vi "RT Main.vi"() -> ()   [LabVIEW 2018]
uses:
  <vilib>/Utility/RT CPU Load.ctl
  <vilib>/FPGAPlugInAG/cRIO-9056/niLvFpga_Open_cRIO-9056.vi
  <vilib>/FPGAPlugInAG/cRIO-9056/niLvFpga_Close_cRIO-9056.vi
  <vilib>/rvi/interface/nirviOpenFPGA/nirviOpenFPGA.xnode
  Type Defs/FPGA reference.ctl
  FPGA Bitfiles/CompressorRigV2_CompressorFPGA_FPGAMainV3_7sPRekuravM.lvbitx
  <vilib>/rvi/interface/nirviCloseFPGA/nirviCloseFPGA.xnode
  <vilib>/NI_Real-Time Target Support.lvlib
panel:
  out "CPU loads":T1[](array[typedef]) {"ISR (%)" format="%#.2f"; "Idle (%)" format="%#.2f"; "Background (%)" format="%#.2f"; "Normal (%)" format="%#.2f"; "Above Normal (%)" format="%#.2f"; "High (%)" format="%#.2g"; "Timed Structures (%)" format="%#.2g"; "Time Critical (%)" format="%#.2g"; "Total (%)" format="%#.2g"}
  in  "Stop display loop":bool
  in  "Queue":enum16{"Message", "Comms", "Data"}(ring)=enum."Data"
  in  "show":bool
  out "messages":string[](array[string])
  out "queue sizes":i32[](array[numeric])
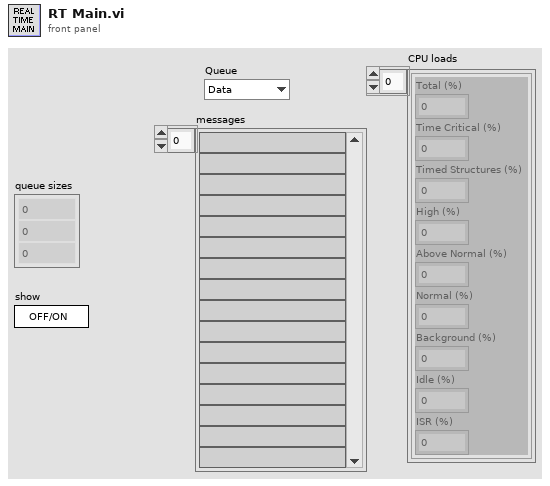
[diagram p1: front panel]
types:
  T1 = typedef "NI_Real-Time Target Support.lvlib/RT CPU Load.ctl" = cluster{"Total (%)":dbl, "Time Critical (%)":dbl, "Timed Structures (%)":dbl, "High (%)":dbl, "Above Normal (%)":dbl, "Normal (%)":dbl, "Background (%)":dbl, "Idle (%)":dbl, "ISR (%)":dbl}
  T2 = typedef "FPGA reference.ctl" = refnum<k20>
  T3 = typedef "Message loop data.ctl" = cluster{"Parameters":cluster{"FPGA Ref":T2, "configID":u32, "activeChannels":cluster{"index":u16, "name":string}[]}, "Variables":cluster{"RT Status":T4, "watchdog":timestamp, "limitsEnabled":bool, "Interlocks":cluster{"gearboxOil":bool, "bearingOil":bool, "gearboxAir":bool}}}
  T4 = typedef "RT Status.ctl" = cluster{"Comms loop":bool, "scheduler loop":bool, "data process loop":bool, "FIFO loop":bool, "Command Stream":bool, "Error Stream":bool, "FPGA FIFO":bool, "Data Stream":bool}
  T5 = typedef "Analogue loop data.ctl" = cluster{"Params":cluster{"FPGA ref":T2, "Total Channels":u32}, "Variables":cluster{"FIFO wait counter":u16, "FIFO read trigger":u32}}
  T6 = typedef "comms data.ctl" = cluster{"Parameters":cluster{"error writer name":string, "command reader name":string, "error buffer size":i32, "command buffer size":i32, "scanivalveIP":string, "scanivalvePeriod":u16}, "Variables":cluster{"listen schedule":u32, "incident buffer":T7[], "command stream":refnum<k21>, "error stream":refnum<k21>, "waiting for command stream connect":bool, "waiting for error stream connect":bool, "scanivalve connection":refnum<k5>, "scanivalveScheduleID":u32, "activeScanivalvePorts":i32[], "channelCount":i16}, "scanivalveConfig":T8}
  T7 = typedef "generic incident.ctl" = cluster{"timestamp":timestamp, "type":string, "Variant":variant}
  T8 = typedef "Scanivalve API.lvlib/scanivalveConfig.ctl" = cluster{"listS":T9, "listC":T10, "listSG":T11, "activeChannels":T12}
  T9 = typedef "Scanivalve API.lvlib/listS.ctl" = cluster{"period":u16, "ADtrig":bool, "ScanTrig":bool, "page":u16, "qpkts":u16}
  T10 = typedef "Scanivalve API.lvlib/listC.ctl" = cluster{"ZC":bool, "unitScan":string, "CvtUnit":dbl, "bin":bool, "EU":bool}
  T11 = typedef "Scanivalve API.lvlib/listSG.ctl" = cluster{"Avg1":u16, "FPS1":u16, "SGEnable1":bool}
  T12 = typedef "Scanivalve API.lvlib/chan1.ctl" = cluster{"Chan1":cluster{"101":bool, "102":bool, "103":bool, "104":bool, "109":bool, "110":bool, "111":bool, "112":bool, "201":bool, "202":bool, "203":bool, "204":bool, "209":bool, "210":bool, "211":bool, "212":bool, "301":bool, "302":bool, "303":bool, "304":bool, "309":bool, "310":bool, "311":bool, "312":bool, "401":bool, "402":bool, "403":bool, "404":bool, "409":bool, "410":bool, "411":bool, "412":bool}}
  T13 = typedef "Data processing loop data.ctl" = cluster{"Parameters":cluster{"FPGA Ref":T2, "data stream":cluster{"data writer name":string, "NS write buffer size":i32, "NS Buffer length":u32}, "FIFO Depth":u32, "Channel controls":cluster{"FIFO channel count":i32, "active indices":i16[], "active channels":i32, "channelScaling":T14[], "scanivalveCount":i32, "channels":refnum<class "Data Channel.lvclass">[]}, "safetyChannels":cluster{"oilP":u16, "airP":u16, "water":u16, "channelLimits":T17[]}, "speedChannel":i32, "maxSpeedLimit":dbl, "Torque":cluster{"fixedOffset":dbl, "filter":bool, "fallingEdge":bool, "swapEncoders":bool}}, "Variables":cluster{"Intermediary buffer":dbl[][], "buffer position":u32, "write loop counter":u16, "NS write trigger":u32, "NS Connection status":bool, "waiting for NS":bool, "labAmbient":cluster{"pressure":dbl, "temperature":dbl}, "scanivalvePorts":u16[], "scanivalvePressures":dbl[], "data stream":refnum<k21>, "activeChannelLimitIndex":u16[], "runningSpeedLimit":dbl, "speedChannelIndex":i32, "Interlocks":cluster{"gearboxOil":bool, "bearingOil":bool, "gearboxAir":bool}, "interlockChannels":cluster{"gearboxOil":i32, "bearingOil":i32, "air":i32}, "limitStates":cluster{"warn":bool, "alarm":bool}[]}}
  T14 = typedef "channelControl.ctl" = cluster{"index":u16, "active":bool, "channelType":T15, "module":u16, "terminal":u16, "channelName":string, "scalingMethod":T16, "scalingParameters":dbl[], "scaledUnits":string, "tempOffset":dbl}
  T15 = typedef "channelScalingTypes.ctl" = enum16{"calculation", "measurement", "scanivalve", "output", "digital"}
  T16 = typedef "scalingMethods.ctl" = enum16{"none", "linear", "thermocouple", "polynomial", "encoder", "RTD"}
  T17 = typedef "channelLimitControl.ctl" = cluster{"channelID":u16, "Enabled":bool, "warnValue":dbl, "limitValue":dbl, "Invert":bool, "limitAction":T18}
  T18 = typedef "limitActions.ctl" = enum16{"stop", "shutdown", "ignore"}
  T19 = cluster{"Message":T3, "FIFO":T5, "Comms data":T6, "Data processor":T13}
  T20 = typedef "Queues cluster.ctl" = cluster{"RT Message":refnum<queue>, "RT Comms":refnum<queue>, "RT Data":refnum<queue>, "RT FIFO":refnum<queue>, "message scheduler":refnum<class "message scheduler.lvclass">}
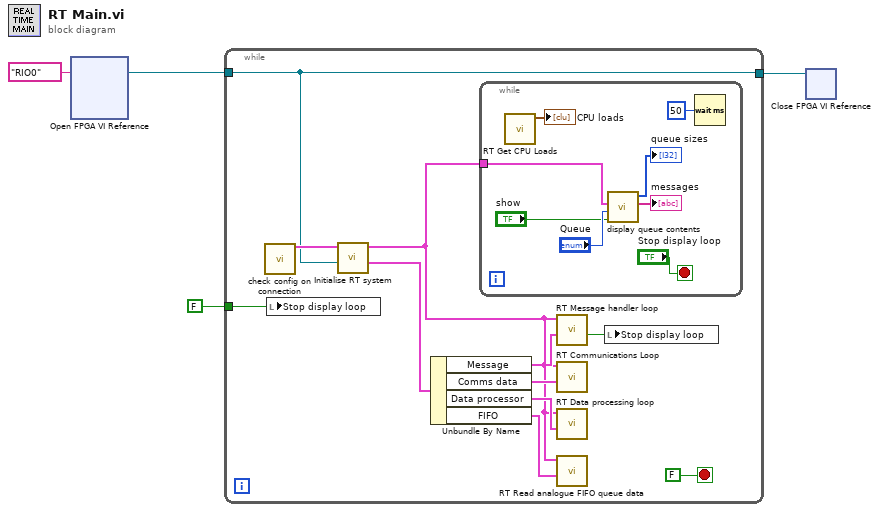
[diagram p0: block diagram]
diagram:
  n1 = xnode "Open FPGA VI Reference"("resource name"=tag "RIO0") -> ("FPGA VI Reference Out"=w3:T2)  [unwired: 1 in, 1 out]
  n2 = while {
    tunnel: w3 -> [w5]
    tunnel: [w5] -> w4
    tunnel: FALSE ("Stop display loop") -> [w6]
    stop <- FALSE stop-if-true
    n3 = call "check config on connection.vi"() -> ("config data out"=w9:T19)  [unwired: 11 in]
    n4 = local write "Stop display loop"(w6) -> ()
    n5 = call "Initialise RT system.vi"("CompressorRigV2"=w5, "config data out"=w9) -> ("config data"=w15:T19, "Queues"=w10:T20)  [unwired: 8 in]
    n6 = Unbundle By Name(w15) -> ("Message"=w14:T3, "Comms data"=w13:T6, "Data processor"=w11:T13, "FIFO"=w12:T5)
    n7 = while {
      tunnel: w10 -> [w23]
      stop <- "Stop display loop" stop-if-true
      n8 = call <vilib>:"RT Get CPU Loads.vi"() -> ("CPU loads"=→"CPU loads":T1[])  [unwired: 10 in, 1 out]
      n9 = call "display queue contents.vi"("show queue contents"="show", "Queue"="Queue", "Queues"=w23) -> ("Array 2"=→"messages":string[], "Queue lengths"=→"queue sizes":i32[])  [unwired: 7 in]
      n10 = Wait (ms)(milliseconds to wait=u32 50) -> ()  [unwired: 1 out]
    }
    n11 = call "RT Message handler loop.vi"("Message handler data"=w14, "RT Queues"=w10) -> ("stop button"=w7:bool)  [unwired: 9 in]
    n12 = call "RT Communications Loop.vi"("Comms data"=w13, "RT Queues"=w10) -> ()  [unwired: 10 in]
    n13 = call "RT Data processing loop.vi"("Data"=w11, "RT Queues"=w10) -> ()  [unwired: 10 in]
    n14 = call "RT Read analogue FIFO queue data.vi"("FIFO parameters"=w12, "RT Queues"=w10) -> ()  [unwired: 10 in]
    n15 = local write "Stop display loop"(w7) -> ()
  }
  n16 = xnode "Close FPGA VI Reference"("FPGA VI Reference In"=w4) -> ()  [unwired: 1 in, 1 out]
